vi "Load Archiving Parameters.vi"(7 "section":string, 8 "error in (no error)":errorcluster, 11 "config ref in":T1) -> (0 "error out":errorcluster, 1 "2 LBCB Archiving Mode":bool, 2 "Log File Size (MBytes)":i64, 3 "Logging Directory":path, 4 "config ref out":T1)   [LabVIEW 2009]
uses:
  <vilib>/Utility/config.llb/Config Data RefNum.ctl
  <vilib>/Utility/config.llb/Read Key (Boolean).vi
  <vilib>/Utility/config.llb/Read Key (U32).vi
  <vilib>/Utility/config.llb/Read Key (Path).vi
  <vilib>/Utility/config.llb/NI_LVConfig.lvlib
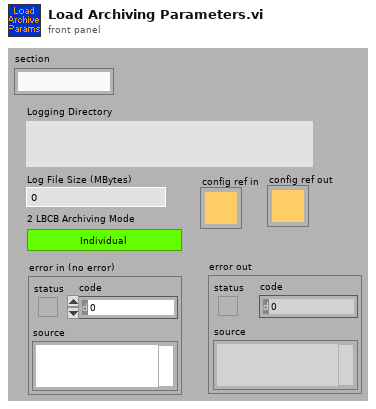
[diagram p1: front panel]
types:
  T1 = typedef "NI_LVConfig.lvlib/Config Data RefNum.ctl" = refnum<k1>
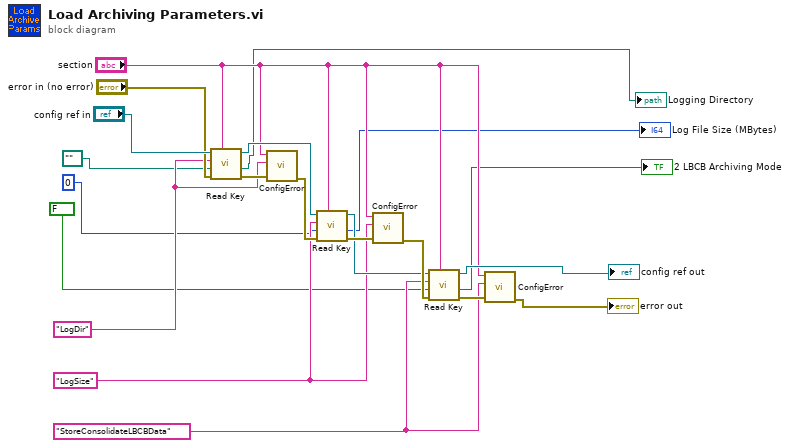
[diagram p0: block diagram]
diagram:
  w7 = "StoreConsolidateLBCBData" ("key")
  w8 = "LogSize" ("key")
  w18 = "LogDir" ("key")
  n1 = call-poly <vilib>:"Read Key.vi"("section"="section", "error in (no error)"="error in (no error)", "default value"=path "" ("Logging Directory"), "key"=w18, "refnum"="config ref in") -> ("error out"=w19:errorcluster, "value"=→"Logging Directory":path, "refnum out"=w12:T1)  [unwired: 3 in, 1 out]
  n2 = call "ConfigError.vi"("error in (no error)"=w19, "Key"=w18, "Section"="section") -> ("error out"=w15:errorcluster)  [unwired: 8 in]
  n3 = call-poly <vilib>:"Read Key.vi"("section"="section", "error in (no error)"=w15, "default value"=i64 0 ("Log File Size (MBytes)"), "key"=w8, "refnum"=w12) -> ("error out"=w17:errorcluster, "value"=→"Log File Size (MBytes)":u32, "refnum out"=w11:T1)  [unwired: 3 in, 1 out]
  n4 = call "ConfigError.vi"("error in (no error)"=w17, "Key"=w8, "Section"="section") -> ("error out"=w14:errorcluster)  [unwired: 8 in]
  n5 = call-poly <vilib>:"Read Key.vi"("section"="section", "error in (no error)"=w14, "default value"=FALSE ("2 LBCB Archiving Mode"), "key"=w7, "refnum"=w11) -> ("error out"=w16:errorcluster, "value"=→"2 LBCB Archiving Mode":bool, "refnum out"=→"config ref out":T1)  [unwired: 3 in, 1 out]
  n6 = call "ConfigError.vi"("error in (no error)"=w16, "Key"=w7, "Section"="section") -> ("error out"=→"error out":errorcluster)  [unwired: 8 in]
